vi "Break out.vi"(8 "error in (no error)":errorcluster caption="错误输入（无错误）", 11 "VISA resource name in":refnum<visa-resource-name> caption="VISA资源名称输入") -> (0 "error out":errorcluster caption="错误输出", 3 "VISA resource name out":refnum<visa-resource-name> caption="VISA资源名称输出")   [LabVIEW 2016]
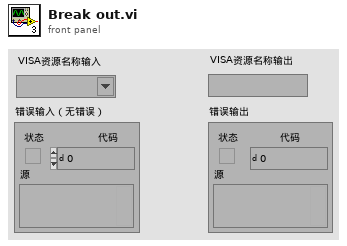
[diagram p1: front panel]
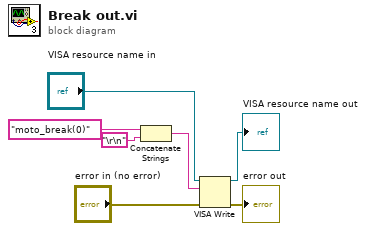
[diagram p0: block diagram]
diagram:
  n1 = Concatenate Strings("moto_break(0)" ("字符串"), "\r\n") -> (w5:string)
  n2 = VISA Write(VISA resource name="VISA resource name in", write buffer=w5, error in (no error)="error in (no error)") -> (VISA resource name out=→"VISA resource name out":refnum<visa-resource-name>, error out=→"error out":errorcluster)  [unwired: 1 out]
